vi "ReceiveWaveform.vi"(8 "error in (no error)":errorcluster, 10 "Waveform":waveform(dbl), 11 "TopUI in":refnum<class "TopUI.lvclass">) -> (0 "error out":errorcluster, 3 "TopUI out":refnum<class "TopUI.lvclass">)   [LabVIEW 2021, in "TopUI.lvlib" / "TopUI.lvclass"]
uses:
  TopUI.lvclass
  TopUI.lvclass/TopUI.ctl
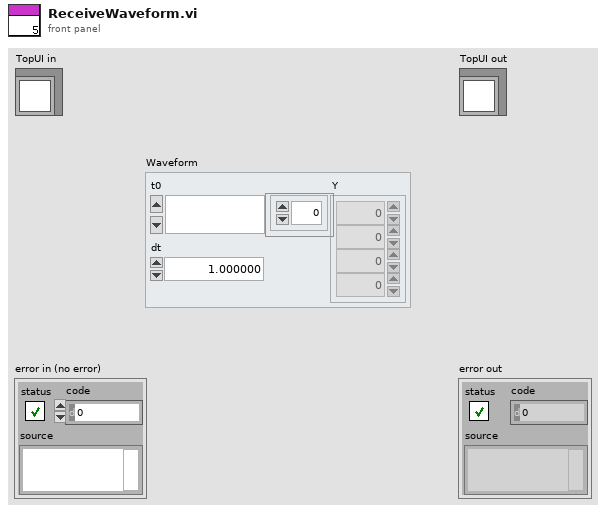
[diagram p1: front panel]
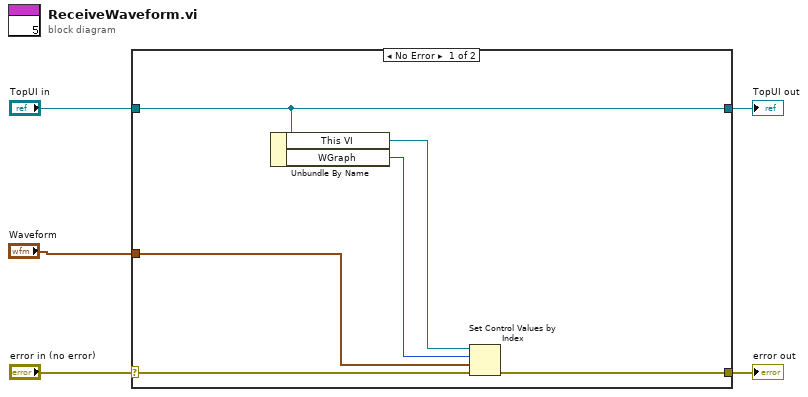
[diagram p0: block diagram]
diagram:
  n1 = case shown="No Error" "error in (no error)" {
    selector: "error in (no error)" -> [w11 w13]
    tunnel: [w10 w13] -> w4
    tunnel: [w9 w12] -> w2
    tunnel: "TopUI in" -> [w9 w12]
    tunnel: "Waveform" -> [w6 _]
    frame No Error {
      n2 = Unbundle By Name(w9) -> ("This VI"=w8:refnum<vi>, "WGraph"=w7:i32)
      n3 = Set Control Values by Index(0:w8, 1:w7, 2:w6, 3:w11) -> (11:w10:errorcluster)
    }
    frame Error {
    }
  }
  "error out" <- w4
  "TopUI out" <- w2
